vi "Extract_Content_from_HTML.vi"(1 "HTML":string) -> (0 "Content":string)   [LabVIEW 2012]
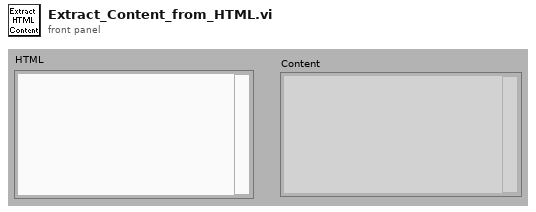
[diagram p1: front panel]
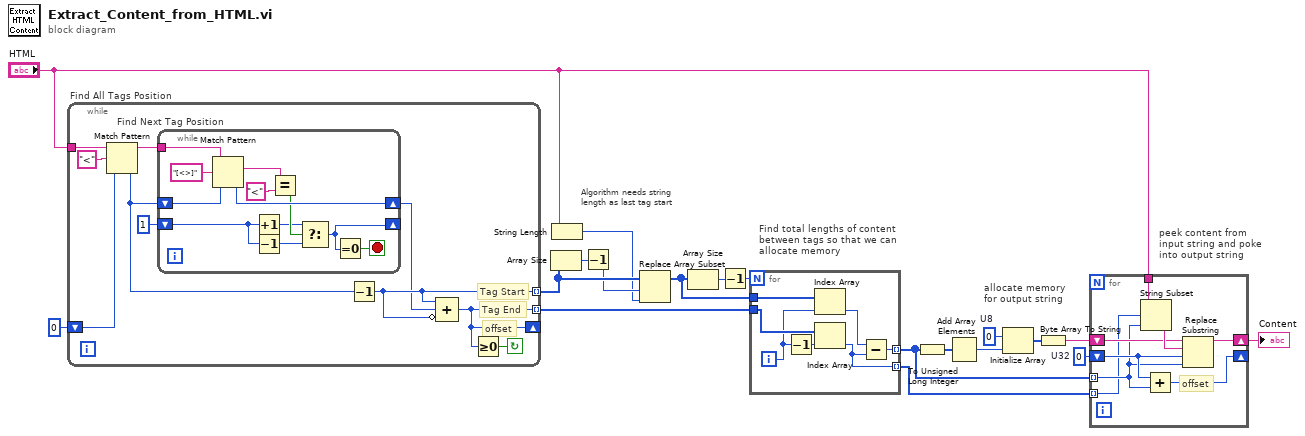
[diagram p0: block diagram]
diagram:
  w11 = u32 0  # U32
  w14 = u8 0  # U8
  # "Find All Tags Position"
  # "peek content from input string and poke into output string"
  # "allocate memory for output string"
  # "Find total lengths of content between tags so that we can allocate memory"
  # "Algorithm needs string length as last tag start"
  n1 = while {
    tunnel: "HTML" -> [w20]
    tunnel: [w24] -> w7 mode=indexing
    tunnel: [w23] -> w1 mode=indexing
    shift-right: [w23] -> _
    shift-left: 0 ("offset (0)") -> [w25]
    stop <- w28 continue-if-true
    # "Find Next Tag Position"
    # "offset"
    # "Tag End"
    # "Tag Start"
    n2 = Match Pattern(string=w20, regular expression="<", offset (0)=w25) -> (offset past match=w22:i32)  [unwired: 3 out]
    n3 = while {
      tunnel: w20 -> [w40]
      shift-right: [w29] -> _
      shift-left: 1 ("offset past match") -> [w33]
      shift-right: [w37] -> w21
      shift-left: w22 -> [w31]
      stop <- w30 stop-if-true
      n4 = Match Pattern(string=w40, regular expression="[<>]", offset (0)=w31) -> (match substring=w38:string, offset past match=w37:i32)  [unwired: 2 out]
      n5 = Increment(x=w33) -> (x+1=w34:i32)
      n6 = Decrement(x=w33) -> (x-1=w32:i32)
      n7 = Equal?(x=w38, y="<") -> (x = y?=w35:bool)
      n8 = Select(t=w34, s=w35, f=w32) -> (s? t:f=w29:i32)
      n9 = Equal To 0?(x=w29) -> (x = 0?=w30:bool)
    }
    n10 = Decrement(x=w22) -> (x-1=w24:i32)
    n11 = Compound Arithmetic op=ADD(w24, w21, invert w24) -> (w23:i32)
    n12 = Greater Or Equal To 0?(x=w23) -> (x >= 0?=w28:bool)
  }
  n13 = Array Size(array=w7) -> (size(s)=w8:i32)
  n14 = String Length(string="HTML") -> (length=w5:i32)
  n15 = Decrement(x=w8) -> (x-1=w6:i32)
  n16 = Replace Array Subset(array=w7, new element=w5, index=w6) -> (w2:i32[])
  n17 = Array Size(array=w2) -> (size(s)=w18:i32)
  n18 = Decrement(x=w18) -> (x-1=w17:i32)
  n19 = for {
    N: w17 -> [_]
    tunnel: w2 -> [w47]
    tunnel: w1 -> [w46]
    tunnel: [w44] -> w4 mode=indexing
    tunnel: [w41] -> w3 mode=indexing
    i -> [w45]
    n20 = Decrement(x=w45) -> (x-1=w43:i32)
    n21 = Index Array(array=w47, index=w45) -> (element=w42:i32)
    n22 = Index Array(array=w46, index=w43) -> (element=w41:i32)
    n23 = Subtract(x=w42, y=w41) -> (x-y=w44:i32)
  }
  n24 = To Unsigned Long Integer(number=w4) -> (unsigned 32bit integer=w16:u32[])
  n25 = Add Array Elements(numeric array=w16) -> (sum=w15:u32)
  n26 = Initialize Array(w14, w15) -> (w13:u8[])
  n27 = Byte Array To String(unsigned byte array=w13) -> (string=w12:string)
  n28 = for {
    shift-right: [w52] -> w10
    shift-left: w12 -> [w53]
    tunnel: "HTML" -> [w55]
    shift-right: [w49] -> _
    shift-left: w11 -> [w51]
    tunnel: w4 -> [w50] mode=indexing
    tunnel: w3 -> [w48] mode=indexing
    # "offset"
    n29 = String Subset(string=w55, offset (0)=w48, length (rest)=w50) -> (substring=w54:string)
    n30 = Add(x=w51, y=w50) -> (x+y=w49:u32)
    n31 = Replace Substring(2:w50, 3:w51, 4:w54, 5:w53) -> (1:w52:string)  [unwired: 1 out]
  }
  "Content" <- w10
